vi "POST (Multipart).vi"(6 "timeout":i32=10000, 7 "output file":path, 8 "error in":errorcluster, 9 "Multipart Post data":T1[](array[typedef]), 10 "url":string, 11 "advanced-http-client in":refnum<class "advanced-http-client.lvclass">) -> (0 "error out":errorcluster, 2 "response":refnum<class "response.lvclass">, 3 "advanced-http-client out":refnum<class "advanced-http-client.lvclass">)   [LabVIEW 2020, in "advanced-http-client.lvclass"]
uses:
  advanced-http-client.lvclass
  advanced-http-client.lvclass/advanced-http-client.ctl
  <vilib>/NI/Advanced HTTP Client/Session.lvclass
  <vilib>/httpClient/MultipartData.ctl
  <vilib>/httpClient/LabVIEWHTTPClient.lvlib
  response/response.lvclass
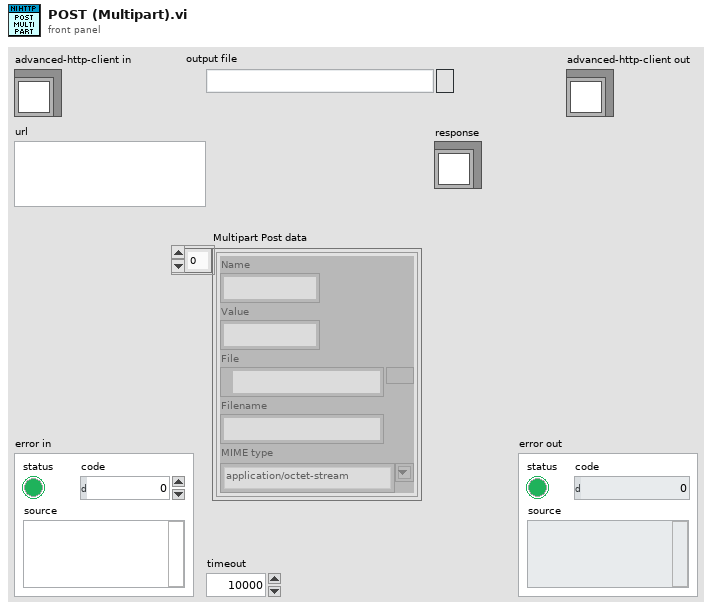
[diagram p1: front panel]
types:
  T1 = typedef "LabVIEWHTTPClient.lvlib/MultipartData.ctl" = cluster{"Name":string, "Value":string, "File":path, "Filename":string, "MIME type":string}
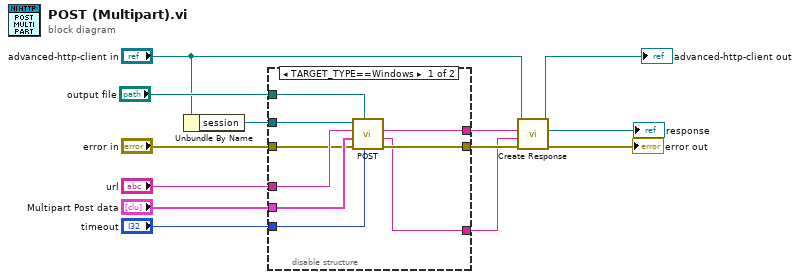
[diagram p0: block diagram]
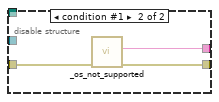
[diagram p2: hidden frame]
diagram:
  n1 = Unbundle By Name("advanced-http-client in") -> ("session"=w13:refnum<class "Session.lvclass">)
  n2 = disable-structure shown="TARGET_TYPE==Windows" {
    disable-tunnel: w13 -> [w22 _]
    disable-tunnel: "url" -> [w21 _]
    disable-tunnel: "Multipart Post data" -> [w20 _]
    disable-tunnel: "error in" -> [w19 w25]
    disable-tunnel: [w18 w24] -> w4
    disable-tunnel: [w17 w23] -> w2
    disable-tunnel: [w16 _] -> w1
    disable-tunnel: "timeout" -> [w15 _]
    disable-tunnel: "output file" -> [w14 _]
    frame condition #0 (active) {
      n3 = call-poly <vilib>:"POST.vi"("timeout"=w15, "output file"=w14, "error in"=w19, "data"=w20, "url"=w21, "session in"=w22) -> ("error out"=w18:errorcluster, "body"=w16:string, "headers"=w17:string)  [unwired: 1 in, 2 out]
    }
    frame condition #1 {
      n4 = call "_os_not_supported.vi"("error in (no error)"=w25) -> ("error out"=w24:errorcluster, "headers"=w23:string)  [unwired: 9 in]
    }
  }
  n5 = call-dynamic "Create Response.vi"("error in (no error)"=w4, "body"=w1, "headers"=w2, "http-client"="advanced-http-client in") -> ("error out"=→"error out":errorcluster, "response"=→"response":refnum<class "response.lvclass">, "http-client out"=→"advanced-http-client out":refnum<class "advanced-http-client.lvclass">)  [unwired: 5 in]
